vi "Write DLL Path.vi"(8 "error in (no error)":errorcluster, 10 "DLL Path":path, 11 "ONNX Class in":refnum<class "ONNX Class.lvclass">) -> (0 "error out":errorcluster, 3 "ONNX Class out":refnum<class "ONNX Class.lvclass">)   [LabVIEW 2017, in "ONNX Class Library.lvlib" / "ONNX Class.lvclass"]
uses:
  ONNX Class.lvclass
  ONNX Class.lvclass/ONNX Class.ctl
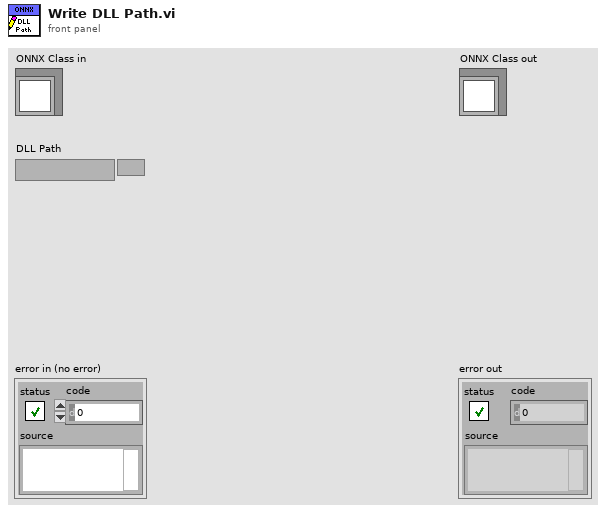
[diagram p1: front panel]
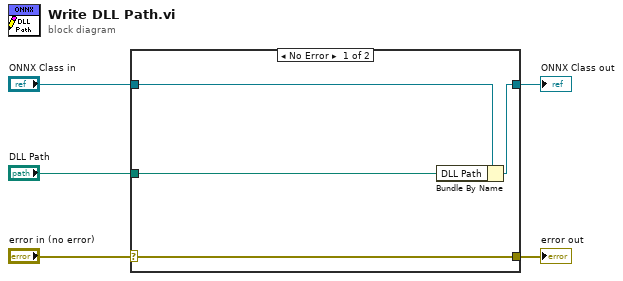
[diagram p0: block diagram]
diagram:
  n1 = case shown="No Error" "error in (no error)" {
    selector: "error in (no error)" -> [w9 w10]
    tunnel: [w9 w10] -> w4
    tunnel: [w7 w11] -> w2
    tunnel: "ONNX Class in" -> [w8 w11]
    tunnel: "DLL Path" -> [w6 _]
    frame No Error {
      n2 = Bundle By Name(cluster=w8, "DLL Path"=w6) -> (w7:refnum<class "ONNX Class.lvclass">)
    }
    frame Error {
    }
  }
  "error out" <- w4
  "ONNX Class out" <- w2
